vi "DisplayMatrixSetting.vi"(8 "error in (no error)":errorcluster, 10 "Measurement":T1(ring), 11 "Pickering in":refnum<class "Pickering.lvclass">) -> (0 "error out":errorcluster, 2 "Display Pickering Matrix":bool[][](array[boolean]), 3 "Pickering out":refnum<class "Pickering.lvclass">)   [LabVIEW 2013, in "Pickering.lvclass"]
uses:
  Pickering.lvclass
  InstrumentSetup.vi
  InstrControl.lvclass
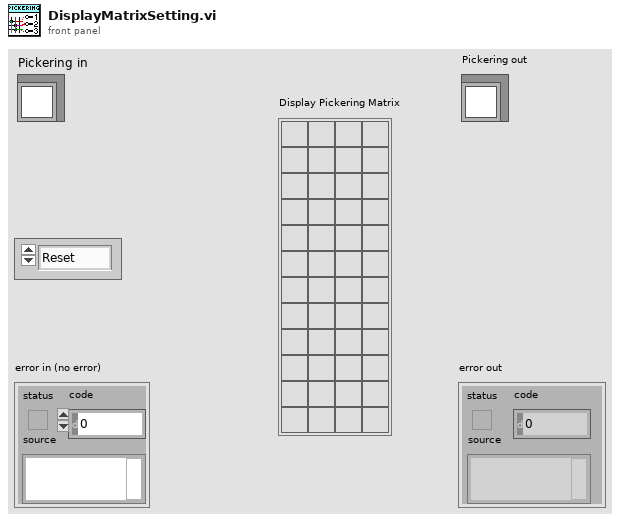
[diagram p1: front panel]
types:
  T1 = enum16{"Reset", "IV", "CV", "Stability", "Striptest", "Cis", "Ris", "PTP"}
  T2 = cluster{"Matrix address":string, "Mux1 address":string, "Mux2 address":string, "Pickering":refnum<class "Pickering.lvclass">, "Matrix X Channels":cluster{"Bias Supply / SMU LO":i32, "Bias Supply / SMU HI":i32, "CV Box LO":i32, "CV Box HI":i32, "CV Box LO IN":i32, "CV Box HI IN":i32, "Volt meter LO":i32, "Volt meter HI":i32, "Mux1 C1":i32, "Mux1 C2":i32, "Mux2 C1":i32, "Mux2 C2":i32}}
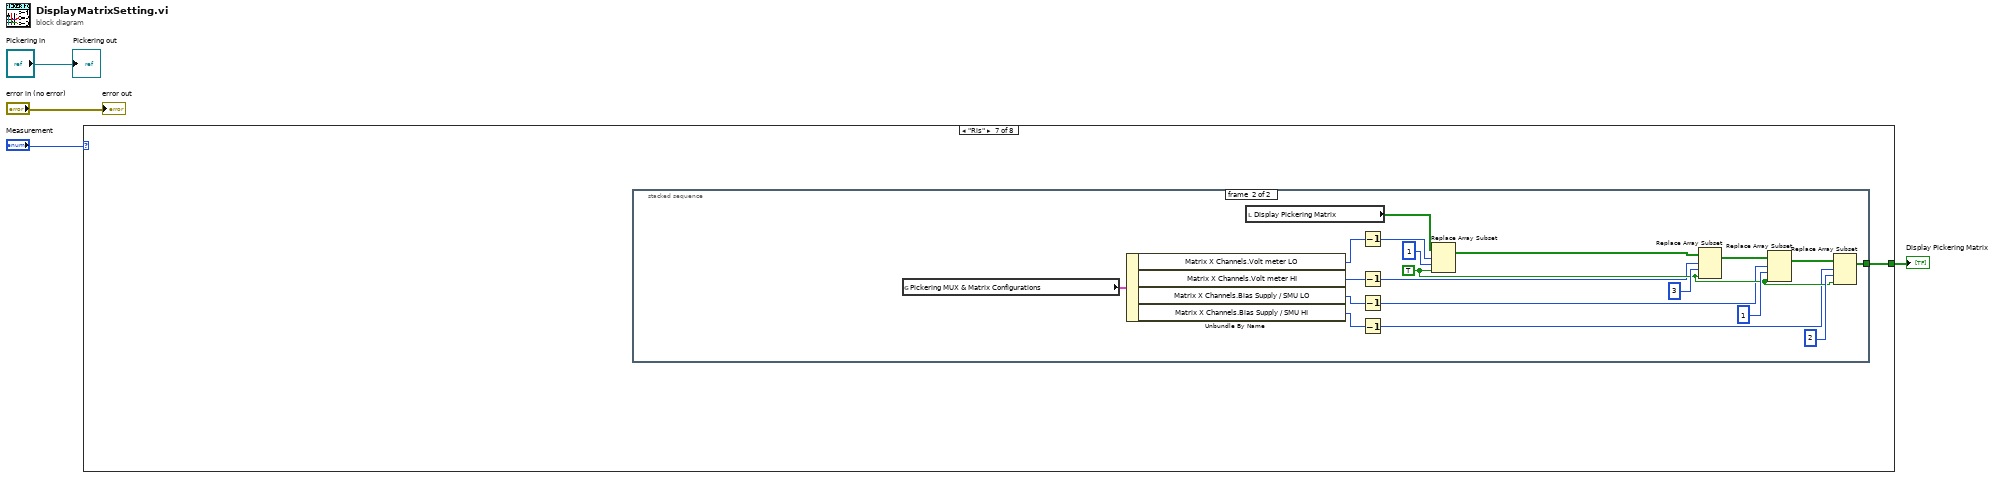
[diagram p0: block diagram]
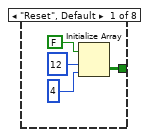
[diagram p2: hidden frame]
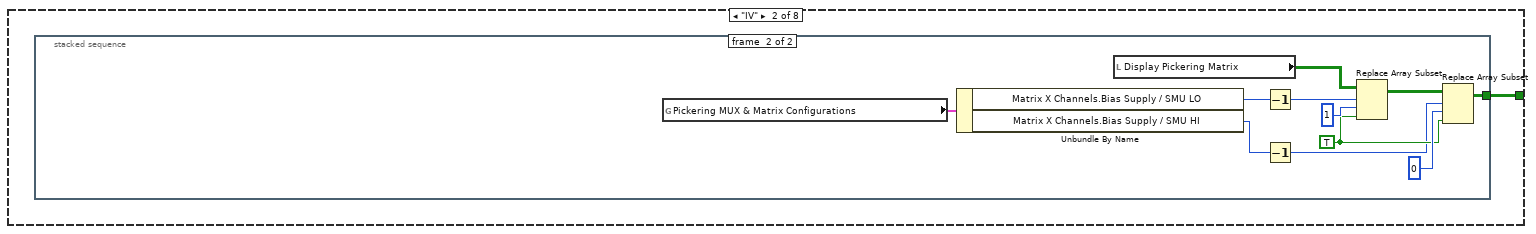
[diagram p3: hidden frame]
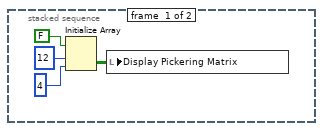
[diagram p4: hidden frame]
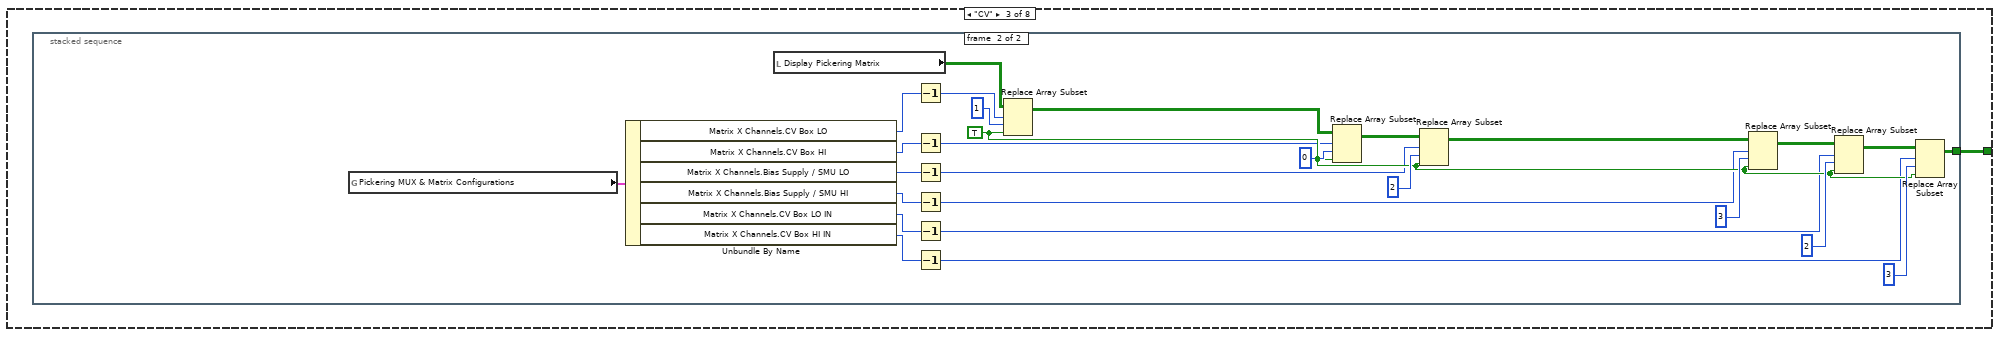
[diagram p5: hidden frame]
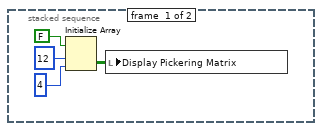
[diagram p6: hidden frame]
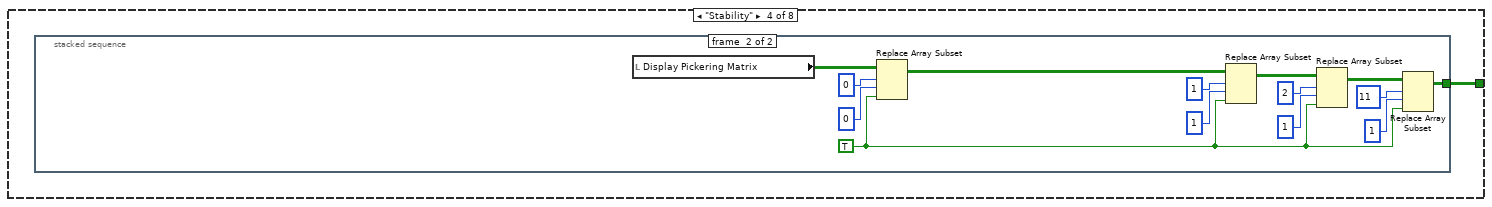
[diagram p7: hidden frame]
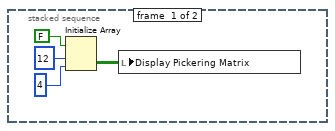
[diagram p8: hidden frame]
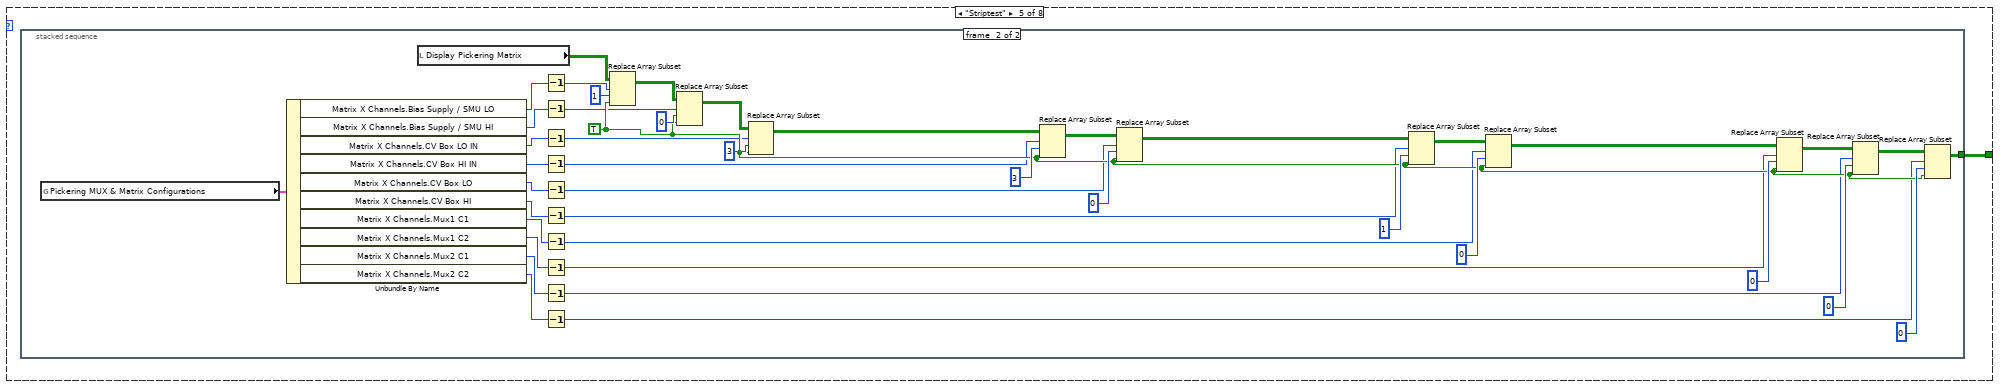
[diagram p9: hidden frame]
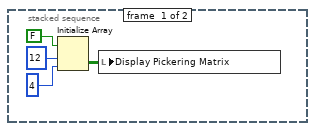
[diagram p10: hidden frame]
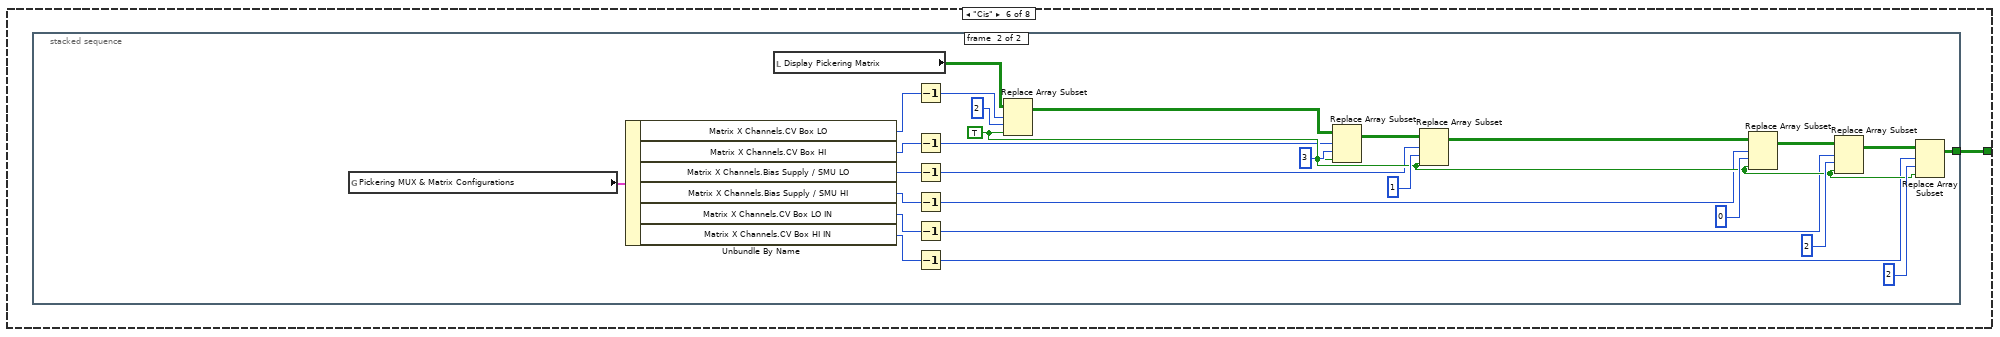
[diagram p11: hidden frame]
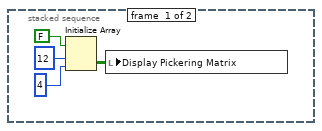
[diagram p12: hidden frame]
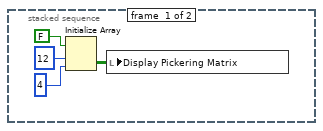
[diagram p13: hidden frame]
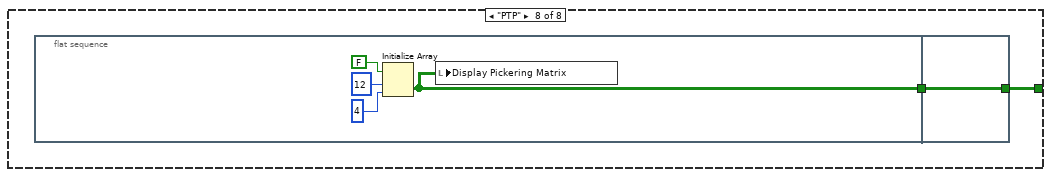
[diagram p14: hidden frame]
diagram:
  n1 = case shown="\"Ris\"" "Measurement" {
    tunnel: [w5 w9 w25 w57 w76 w124 w156 w180] -> w3
    frame "Reset", Default {
      n2 = Initialize Array(FALSE, 12, 4) -> (w5:bool[][])
    }
    frame "IV" {
      n3 = stacked-sequence {
        tunnel: [_ w19] -> w9
        frame #0 {
          n4 = Initialize Array(FALSE, 12, 4) -> (w11:bool[][])
          n5 = local write "Display Pickering Matrix"(w11) -> ()
        }
        frame #1 {
          w21 = TRUE
          n6 = global read "InstrumentSetup.vi" "Pickering MUX & Matrix Configurations"() -> (w18:T2)
          n7 = Unbundle By Name(w18) -> ("Matrix X Channels.Bias Supply / SMU LO"=w17:i32, "Matrix X Channels.Bias Supply / SMU HI"=w16:i32)
          n8 = local read "Display Pickering Matrix"() -> (w20:bool[][])
          n9 = Decrement(x=w17) -> (x-1=w14:i32)
          n10 = Decrement(x=w16) -> (x-1=w15:i32)
          n11 = Replace Array Subset(array=w20, new element=w21, index (row)=w14, index (col)=1) -> (w22:bool[][])
          n12 = Replace Array Subset(array=w22, new element=w21, index (row)=w15, index (col)=0) -> (w19:bool[][])
        }
      }
    }
    frame "CV" {
      n13 = stacked-sequence {
        tunnel: [_ w43] -> w25
        frame #0 {
          n14 = Initialize Array(FALSE, 12, 4) -> (w27:bool[][])
          n15 = local write "Display Pickering Matrix"(w27) -> ()
        }
        frame #1 {
          w45 = TRUE
          n16 = global read "InstrumentSetup.vi" "Pickering MUX & Matrix Configurations"() -> (w42:T2)
          n17 = Unbundle By Name(w42) -> ("Matrix X Channels.CV Box LO"=w41:i32, "Matrix X Channels.CV Box HI"=w36:i32, "Matrix X Channels.Bias Supply / SMU LO"=w37:i32, "Matrix X Channels.Bias Supply / SMU HI"=w38:i32, "Matrix X Channels.CV Box LO IN"=w39:i32, "Matrix X Channels.CV Box HI IN"=w40:i32)
          n18 = local read "Display Pickering Matrix"() -> (w44:bool[][])
          n19 = Decrement(x=w41) -> (x-1=w35:i32)
          n20 = Decrement(x=w36) -> (x-1=w34:i32)
          n21 = Decrement(x=w37) -> (x-1=w33:i32)
          n22 = Decrement(x=w38) -> (x-1=w32:i32)
          n23 = Decrement(x=w39) -> (x-1=w31:i32)
          n24 = Decrement(x=w40) -> (x-1=w30:i32)
          n25 = Replace Array Subset(array=w44, new element=w45, index (row)=w35, index (col)=1) -> (w54:bool[][])
          n26 = Replace Array Subset(array=w54, new element=w45, index (row)=w34, index (col)=0) -> (w53:bool[][])
          n27 = Replace Array Subset(array=w53, new element=w45, index (row)=w33, index (col)=2 ("Index")) -> (w52:bool[][])
          n28 = Replace Array Subset(array=w52, new element=w45, index (row)=w32, index (col)=3 ("Index")) -> (w46:bool[][])
          n29 = Replace Array Subset(array=w46, new element=w45, index (row)=w31, index (col)=2) -> (w47:bool[][])
          n30 = Replace Array Subset(array=w47, new element=w45, index (row)=w30, index (col)=3) -> (w43:bool[][])
        }
      }
    }
    frame "Stability" {
      n31 = stacked-sequence {
        tunnel: [_ w62] -> w57
        frame #0 {
          n32 = Initialize Array(FALSE, 12, 4) -> (w59:bool[][])
          n33 = local write "Display Pickering Matrix"(w59) -> ()
        }
        frame #1 {
          w63 = TRUE
          n34 = local read "Display Pickering Matrix"() -> (w75:bool[][])
          n35 = Replace Array Subset(array=w75, new element=w63, index (row)=0, index (col)=0) -> (w72:bool[][])
          n36 = Replace Array Subset(array=w72, new element=w63, index (row)=1, index (col)=1) -> (w65:bool[][])
          n37 = Replace Array Subset(array=w65, new element=w63, index (row)=2, index (col)=1) -> (w64:bool[][])
          n38 = Replace Array Subset(array=w64, new element=w63, index (row)=11, index (col)=1) -> (w62:bool[][])
        }
      }
    }
    frame "Striptest" {
      n39 = stacked-sequence {
        tunnel: [_ w102] -> w76
        frame #0 {
          n40 = Initialize Array(FALSE, 12, 4) -> (w78:bool[][])
          n41 = local write "Display Pickering Matrix"(w78) -> ()
        }
        frame #1 {
          w104 = TRUE
          n42 = global read "InstrumentSetup.vi" "Pickering MUX & Matrix Configurations"() -> (w101:T2)
          n43 = Unbundle By Name(w101) -> ("Matrix X Channels.Bias Supply / SMU LO"=w100:i32, "Matrix X Channels.Bias Supply / SMU HI"=w95:i32, "Matrix X Channels.CV Box LO IN"=w96:i32, "Matrix X Channels.CV Box HI IN"=w97:i32, "Matrix X Channels.CV Box LO"=w98:i32, "Matrix X Channels.CV Box HI"=w99:i32, "Matrix X Channels.Mux1 C1"=w91:i32, "Matrix X Channels.Mux1 C2"=w92:i32, "Matrix X Channels.Mux2 C1"=w93:i32, "Matrix X Channels.Mux2 C2"=w94:i32)
          n44 = local read "Display Pickering Matrix"() -> (w112:bool[][])
          n45 = Decrement(x=w100) -> (x-1=w90:i32)
          n46 = Decrement(x=w95) -> (x-1=w89:i32)
          n47 = Decrement(x=w96) -> (x-1=w88:i32)
          n48 = Decrement(x=w97) -> (x-1=w87:i32)
          n49 = Decrement(x=w98) -> (x-1=w86:i32)
          n50 = Decrement(x=w99) -> (x-1=w85:i32)
          n51 = Decrement(x=w91) -> (x-1=w84:i32)
          n52 = Decrement(x=w92) -> (x-1=w83:i32)
          n53 = Decrement(x=w93) -> (x-1=w82:i32)
          n54 = Decrement(x=w94) -> (x-1=w81:i32)
          n55 = Replace Array Subset(array=w112, new element=w104, index (row)=w90, index (col)=1) -> (w121:bool[][])
          n56 = Replace Array Subset(array=w121, new element=w104, index (row)=w89, index (col)=0) -> (w120:bool[][])
          n57 = Replace Array Subset(array=w120, new element=w104, index (row)=w88, index (col)=3 ("Index")) -> (w119:bool[][])
          n58 = Replace Array Subset(array=w119, new element=w104, index (row)=w87, index (col)=3 ("Index")) -> (w113:bool[][])
          n59 = Replace Array Subset(array=w113, new element=w104, index (row)=w86, index (col)=0) -> (w114:bool[][])
          n60 = Replace Array Subset(array=w114, new element=w104, index (row)=w85, index (col)=1) -> (w103:bool[][])
          n61 = Replace Array Subset(array=w103, new element=w104, index (row)=w84, index (col)=0) -> (w107:bool[][])
          n62 = Replace Array Subset(array=w107, new element=w104, index (row)=w83, index (col)=0) -> (w106:bool[][])
          n63 = Replace Array Subset(array=w106, new element=w104, index (row)=w82, index (col)=0) -> (w105:bool[][])
          n64 = Replace Array Subset(array=w105, new element=w104, index (row)=w81, index (col)=0) -> (w102:bool[][])
        }
      }
    }
    frame "Cis" {
      n65 = stacked-sequence {
        tunnel: [_ w129] -> w124
        frame #0 {
          n66 = Initialize Array(FALSE, 12, 4) -> (w126:bool[][])
          n67 = local write "Display Pickering Matrix"(w126) -> ()
        }
        frame #1 {
          w145 = TRUE
          n68 = global read "InstrumentSetup.vi" "Pickering MUX & Matrix Configurations"() -> (w144:T2)
          n69 = Unbundle By Name(w144) -> ("Matrix X Channels.CV Box LO"=w143:i32, "Matrix X Channels.CV Box HI"=w138:i32, "Matrix X Channels.Bias Supply / SMU LO"=w139:i32, "Matrix X Channels.Bias Supply / SMU HI"=w140:i32, "Matrix X Channels.CV Box LO IN"=w141:i32, "Matrix X Channels.CV Box HI IN"=w142:i32)
          n70 = local read "Display Pickering Matrix"() -> (w135:bool[][])
          n71 = Decrement(x=w143) -> (x-1=w137:i32)
          n72 = Decrement(x=w138) -> (x-1=w136:i32)
          n73 = Decrement(x=w139) -> (x-1=w133:i32)
          n74 = Decrement(x=w140) -> (x-1=w132:i32)
          n75 = Decrement(x=w141) -> (x-1=w131:i32)
          n76 = Decrement(x=w142) -> (x-1=w130:i32)
          n77 = Replace Array Subset(array=w135, new element=w145, index (row)=w137, index (col)=2) -> (w146:bool[][])
          n78 = Replace Array Subset(array=w146, new element=w145, index (row)=w136, index (col)=3) -> (w134:bool[][])
          n79 = Replace Array Subset(array=w134, new element=w145, index (row)=w133, index (col)=1) -> (w153:bool[][])
          n80 = Replace Array Subset(array=w153, new element=w145, index (row)=w132, index (col)=0) -> (w152:bool[][])
          n81 = Replace Array Subset(array=w152, new element=w145, index (row)=w131, index (col)=2 ("Index")) -> (w151:bool[][])
          n82 = Replace Array Subset(array=w151, new element=w145, index (row)=w130, index (col)=2 ("Index")) -> (w129:bool[][])
        }
      }
    }
    frame "Ris" {
      n83 = stacked-sequence {
        tunnel: [_ w170] -> w156
        frame #0 {
          n84 = Initialize Array(FALSE, 12, 4) -> (w158:bool[][])
          n85 = local write "Display Pickering Matrix"(w158) -> ()
        }
        frame #1 {
          w171 = TRUE
          n86 = global read "InstrumentSetup.vi" "Pickering MUX & Matrix Configurations"() -> (w169:T2)
          n87 = Unbundle By Name(w169) -> ("Matrix X Channels.Volt meter LO"=w168:i32, "Matrix X Channels.Volt meter HI"=w165:i32, "Matrix X Channels.Bias Supply / SMU LO"=w166:i32, "Matrix X Channels.Bias Supply / SMU HI"=w167:i32)
          n88 = local read "Display Pickering Matrix"() -> (w179:bool[][])
          n89 = Decrement(x=w168) -> (x-1=w161:i32)
          n90 = Decrement(x=w165) -> (x-1=w162:i32)
          n91 = Decrement(x=w166) -> (x-1=w164:i32)
          n92 = Decrement(x=w167) -> (x-1=w163:i32)
          n93 = Replace Array Subset(array=w179, new element=w171, index (row)=w161, index (col)=1) -> (w177:bool[][])
          n94 = Replace Array Subset(array=w177, new element=w171, index (row)=w162, index (col)=3) -> (w174:bool[][])
          n95 = Replace Array Subset(array=w174, new element=w171, index (row)=w164, index (col)=1) -> (w172:bool[][])
          n96 = Replace Array Subset(array=w172, new element=w171, index (row)=w163, index (col)=2) -> (w170:bool[][])
        }
      }
    }
    frame "PTP" {
      n97 = flat-sequence {
        tunnel: [w182] -> w181
        tunnel: w181 -> [w186]
        tunnel: [w186] -> w180
        frame #0 {
          n98 = Initialize Array(FALSE, 12, 4) -> (w182:bool[][])
          n99 = local write "Display Pickering Matrix"(w182) -> ()
        }
        frame #1 {
        }
      }
    }
  }
  "Display Pickering Matrix" <- w3
  "Pickering out" <- "Pickering in"
  "error out" <- "error in (no error)"
